vi "histogram grab.vi"() -> ()   [LabVIEW 2013]
uses:
  <vilib>/vision/NI_Vision_Development_Module.lvlib
panel:
  out "histogram":T1(graph)
  out "ms between image":u32
  out "Frame Rate":dbl
  in  "Stop (F)":bool
  out "Image Out":T2(plugin-control)
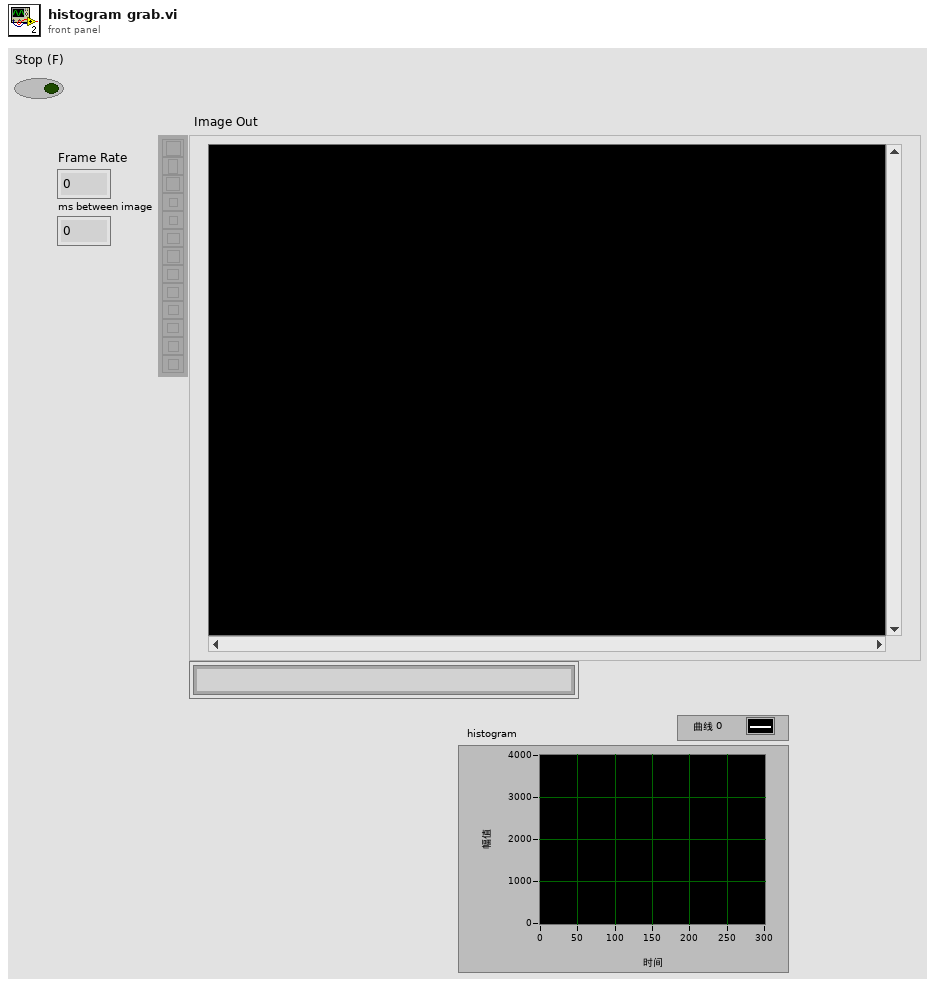
[diagram p1: front panel]
types:
  T1 = cluster{"Starting Value":sgl, "Incremental Value":sgl, "Histogram":u32[]}
  T2 = typedef "IMAQ Image.ctl" = refnum<image>
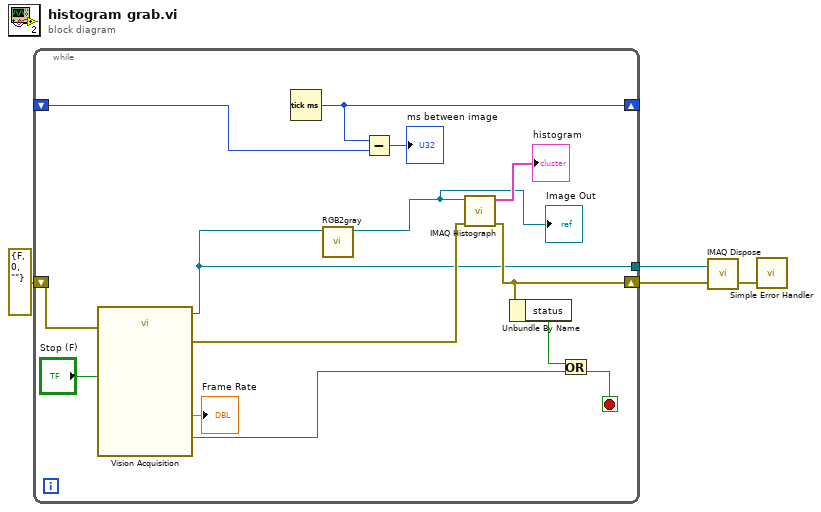
[diagram p0: block diagram]
diagram:
  n1 = while {
    shift-right: [w15] -> _
    shift-left: _ -> [w14]
    shift-right: [w8] -> w4
    shift-left: errorcluster {"status"=FALSE, "code"=0, "source"=""} ("error out") -> [w11]
    tunnel: [w6] -> w2
    stop <- w12 stop-if-true
    n2 = call "Vision Acquisition"("Stop (F)"="Stop (F)", "error in"=w11) -> ("Image Out"=w6:T2, "Frame Rate"=→"Frame Rate":dbl, "Stopped"=w17:bool, "error out"=w9:errorcluster)  [unwired: 22 in]
    n3 = Tick Count (ms)() -> (millisecond timer value=w15:u32)
    n4 = call "RGB2gray.vi"("引用句柄输入"=w6) -> ("引用句柄输出"=w5:T2)  [unwired: 10 in]
    "Image Out" <- w5
    n5 = Subtract(x=w15, y=w14) -> (x-y=→"ms between image":u32)
    n6 = call "IMAQ Histograph"("error in (no error)"=w9, "Image"=w5) -> ("error out"=w8:errorcluster, "Histogram Graph"=→"histogram":T1)  [unwired: 6 in, 2 out]
    n7 = Unbundle By Name(w8) -> ("status"=w10:bool)
    n8 = Or(x=w10, y=w17) -> (x .or. y?=w12:bool)
  }
  n9 = call "IMAQ Dispose"("Image"=w2, "error in (no error)"=w4) -> ("error out"=w1:errorcluster)  [unwired: 4 in]
  n10 = call <vilib>:"Simple Error Handler.vi"("error in (no error)"=w1) -> ()  [unwired: 4 in, 5 out]
